vi "Sparse_Coded_Signal.vi"(8 "error in (no error)":errorcluster caption="entrée d'erreur (pas d'erreur)", 11 "make_sparse_coded_signal":T2={"n_samples"=100, "n_components"=1, "n_features"=5, " n_nonzero_coefs"=1, "random_state"=-1, "Returns"="data"} {"random_state" min=-1; "n_features" min=1; "n_samples" min=1}) -> (0 "error out":errorcluster, 3 "Data":T1)   [LabVIEW 2020]
doc: "Generate a signal as a sparse combination of dictionary elements.\n\nReturns a matrix Y = DX, such as D is (n_features, n_components), X is (n_components, n_samples) and each column of X has exactly n_nonzero_coefs non-zero elements. \n\n\n\n\nParameters :\n\n- n_samples : int\nnumber of samples to generate\n\n- n_components : int,\nnumber of components in the dictionary\n\n- n_features : int\nnumber of features of the dataset to generate\n\n- n_nonzero_coefs : int\nnumber of active (non-zero) coefficients in each sample\n\n- random_state : int, RandomState instance, default=None=-1\nDetermines random number generation for dataset creation. Pass an int for reproducible output across multiple function calls. See Glossary.\n\nReturns : \n\n- data : array of shape [n_features, n_samples]\nThe encoded signal (Y).\n\n- dictionary : array of shape [n_features, n_components]\nThe dictionary with normalized components (D).\n\n- code : array of shape [n_components, n_samples]\nThe sparse code such that each column of this matrix has exactly n_nonzero_coefs non-zero items (X)."
uses:
  Sparse_Coded_Signal.lvclass
panel:
  out "Sparse_Coded_Signal.lvclass":refnum<class "Sparse_Coded_Signal.lvclass">
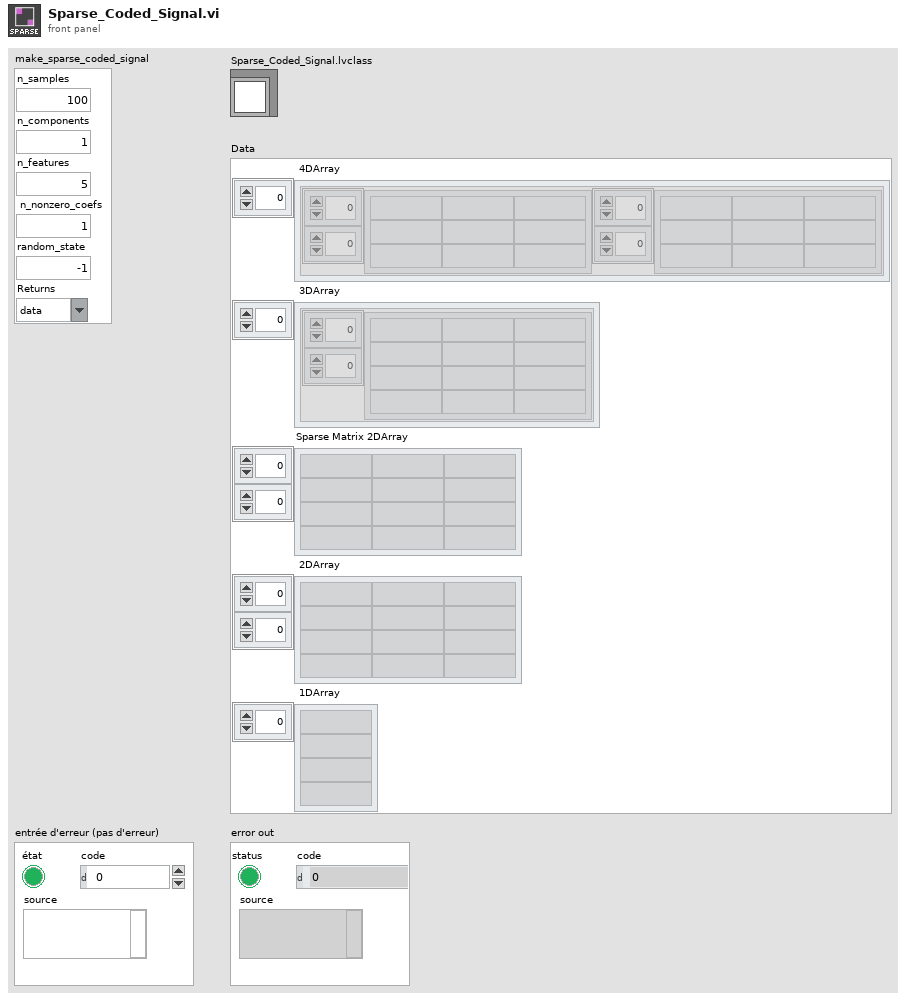
[diagram p1: front panel]
types:
  T1 = cluster{" 4DArray":cluster{"1":string[][], "2":string[][]}[], " 3DArray":cluster{"Tableau":string[][]}[], "Sparse Matrix 2DArray":string[][], " 2DArray":string[][], " 1DArray":string[]}
  T2 = cluster{"n_samples":u32, "n_components":u32, "n_features":u32, " n_nonzero_coefs":u32, "random_state":i32, "Returns":string}
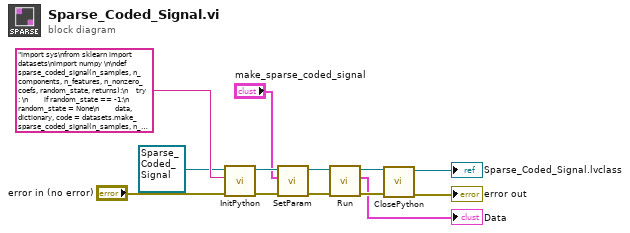
[diagram p0: block diagram]
diagram:
  n1 = call-dynamic "InitPython.vi"("error in (no error)"="error in (no error)", "Python Instruction"="import sys\nfrom sklearn import datasets\nimport numpy \n\ndef sparse_coded_signal(n_samples, n_components, n_features, n_nonzero_coefs, random_state, returns):\n    try : \n        if random_state == -1:\n            random_state = None\n        data, dictionary, code = datasets.make_sparse_coded_signal(n_samples, n_components, n_features, n_nonzero_coefs, random_state)\n        if returns == 'data':\n            datalist = data.tolist()\n            return str(datalist)\n        elif returns == 'dictionary':\n            datalist = dictionary.tolist()\n            return str(datalist)\n        else:\n            datalist = code.tolist()\n            return str(datalist)\n    except:\n        erreur = sys.exc_info()\n        typerr = u\"%s\" % (erreur[0])\n        typerr = typerr[typerr.find(\"'\")+1:typerr.rfind(\"'\")]\n        msgerr = u\"%s\" % (erreur[1])\n        message = str('/!\\\\ {0} : {1}'. format(typerr,msgerr))\n        return message", "Scikit-learn en entrée"=refnum<class "Sparse_Coded_Signal.lvclass"> refnum ("Sparse_Coded_Signal.lvclass")) -> ("error out"=w8:errorcluster, "Scikit-learn en sortie"=w10:refnum<class "Sparse_Coded_Signal.lvclass">)  [unwired: 7 in]
  n2 = call-dynamic "SetParam.vi"("error in (no error)"=w8, "make_sparse_coded_signal"="make_sparse_coded_signal", "Sparse_Coded_Signal.lvclass"=w10) -> ("error out"=w6:errorcluster, "Sparse_Coded_Signal.lvclass"=w7:refnum<class "Sparse_Coded_Signal.lvclass">)  [unwired: 7 in]
  n3 = call-dynamic "Run.vi"("error in (no error)"=w6, "Sparse_Coded_Signal.lvclass"=w7) -> ("error out"=w4:errorcluster, "Data"=→"Data":T1, "Sparse_Coded_Signal.lvclass"=w5:refnum<class "Sparse_Coded_Signal.lvclass">)  [unwired: 7 in]
  n4 = call-dynamic "ClosePython.vi"("error in (no error)"=w4, "Scikit-learn en entrée"=w5) -> ("error out"=→"error out":errorcluster, "Scikit-learn en sortie"=→"Sparse_Coded_Signal.lvclass":refnum<class "Sparse_Coded_Signal.lvclass">)  [unwired: 8 in]
